vi "GetParam.vi"(8 "error in (no error)":errorcluster caption="entrée d'erreur (pas d'erreur)", 11 "Paired_distances.lvclass":refnum<class "Paired_distances.lvclass">) -> (0 "error out":errorcluster caption="sortie d'erreur", 2 "paired_distances":cluster{"metric":string}={"metric"="euclidean"}, 3 "Paired_distances.lvclass":refnum<class "Paired_distances.lvclass">)   [LabVIEW 2020, in "Paired_distances.lvclass"]
doc: "Get Parameters"
uses:
  Paired_distances.lvclass
  Paired_distances.lvclass/Paired_distances.ctl
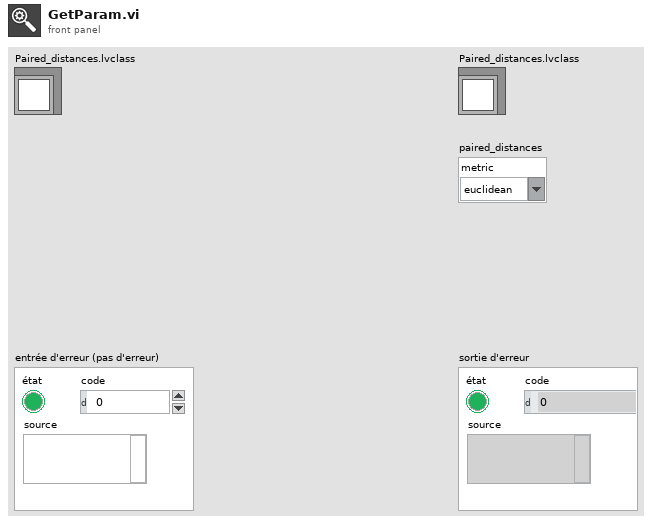
[diagram p1: front panel]
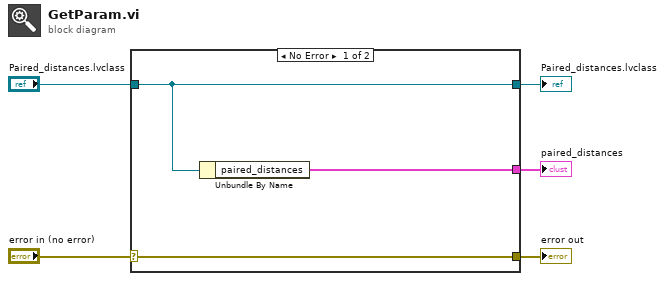
[diagram p0: block diagram]
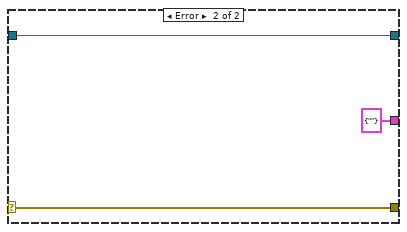
[diagram p2: hidden frame]
diagram:
  n1 = case shown="No Error" "error in (no error)" {
    selector: "error in (no error)" -> [w8 w10]
    tunnel: [w8 w10] -> w4
    tunnel: [w7 w11] -> w2
    tunnel: "Paired_distances.lvclass" -> [w7 w11]
    tunnel: [w6 cluster{"metric":string} {"metric"=""} ("paired_distances")] -> w1
    frame No Error {
      n2 = Unbundle By Name(w7) -> ("paired_distances"=w6:cluster{"metric":string})
    }
    frame Error {
    }
  }
  "error out" <- w4
  "Paired_distances.lvclass" <- w2
  "paired_distances" <- w1
